vi "Do.vi"(8 "error in (no error)":errorcluster, 10 "Actor in":refnum<class "Actor.lvclass">, 11 "Unregister by Name Msg in":refnum<class "Unregister by Name Msg.lvclass">) -> (0 "error out":errorcluster, 2 "Actor out":refnum<class "Actor.lvclass">)   [LabVIEW 2023, in "MVC Actors.lvlib" / "Unregister by Name Msg.lvclass"]
doc: "(<B>Filename</B>: Actor Framework.lvlib:Message.lvclass:Do.vi)\n\nDefines what a message does when it is received by an actor. Generally, a message instructs an actor to invoke one of its methods. By default, this method does nothing. A child class must override it to define behavior. Create a child class by using the Actor Framework Message Maker dialog box."
uses:
  Unregister by Name Msg.lvclass
  Unregister by Name Msg.lvclass/Unregister by Name Msg.ctl
  Controller/Controller.lvclass
  C:/Program Files/National Instruments/LabVIEW 2023/vi.lib/LS Instruments AG/Async Methods Actor/Async Methods Actor/Async Methods Actor/Async Methods Actor.lvclass
  C:/Program Files/National Instruments/LabVIEW 2023/vi.lib/ActorFramework/Actor/Actor.lvclass
  C:/Projects/Shared Libraries/Event Actors/Controller/Controller.lvclass
  <vilib>/ActorFramework/Actor/Actor.lvclass
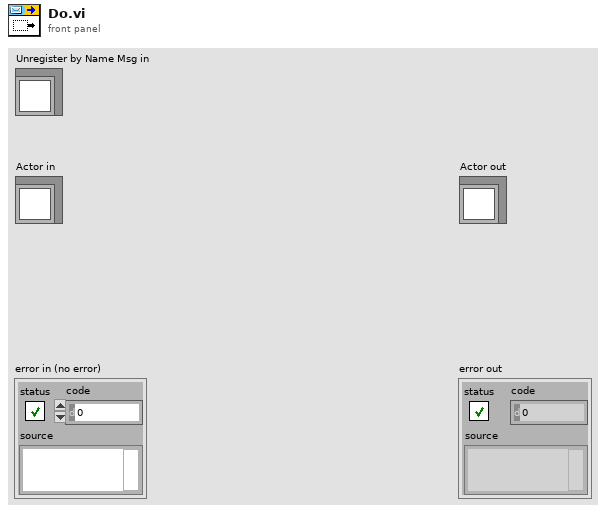
[diagram p1: front panel]
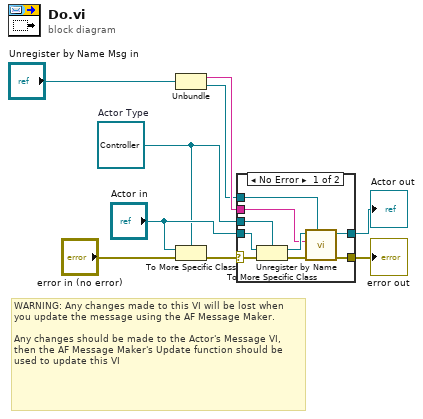
[diagram p0: block diagram]
diagram:
  w4 = refnum<class "Controller.lvclass"> refnum  # Actor Type
  # "WARNING: Any changes made to this VI will be lost when you update the message using the AF Message Maker.\n\nAny changes should be made to the Actor's Message VI, then the AF Message Maker's Update function should be used to update this VI"
  n1 = Unbundle("Unregister by Name Msg in") -> (w3:string, w2:refnum<class "Event.lvclass">)
  n2 = To More Specific Class(target class=w4, reference="Actor in", error in="error in (no error)") -> (error out=w8:errorcluster)  [unwired: 1 out]
  n3 = case shown="No Error" w8 {
    selector: w8 -> [w18 w20]
    tunnel: [w13 w20] -> w7
    tunnel: [w12 w19] -> w6
    tunnel: "Actor in" -> [w17 w19]
    tunnel: w4 -> [w16 _]
    tunnel: w3 -> [w11 _]
    tunnel: w2 -> [w10 _]
    frame No Error {
      n4 = To More Specific Class ("Actor Cast")(target class=w16, reference=w17, error in=w18) -> (specific class reference=w15:refnum<class "Controller.lvclass">, error out=w14:errorcluster)
      n5 = call "Unregister by Name.vi"("Event"=w10, "error in (no error)"=w14, "View Name"=w11, "Controller in"=w15) -> ("error out"=w13:errorcluster, "Controller out"=w12:refnum<class "Controller.lvclass">)  [unwired: 6 in]
    }
    frame Error {
    }
  }
  "error out" <- w7
  "Actor out" <- w6
